vi "Get Positions.vi"(8 "error in":errorcluster, 11 "Stage VISA in":refnum<visa-resource-name>) -> (0 "error out":errorcluster, 2 "Stage current position":dbl[](array[numeric]), 3 "Stage VISA out":refnum<visa-resource-name>)   [LabVIEW 2017]
panel:
  # "X"
  # "Y"
  # "Z"
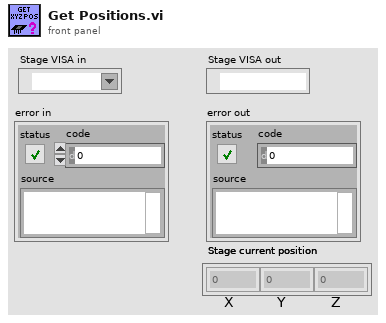
[diagram p1: front panel]
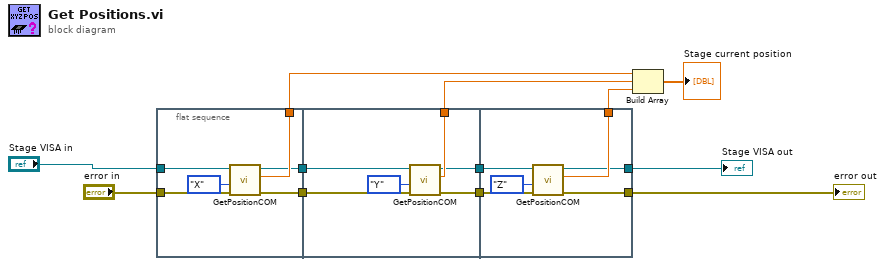
[diagram p0: block diagram]
diagram:
  n1 = flat-sequence {
    tunnel: "error in" -> [w17]
    tunnel: [w18] -> w10
    tunnel: [w16] -> w7
    tunnel: [w15] -> w3
    tunnel: "Stage VISA in" -> [w14]
    tunnel: [w22] -> w6
    tunnel: [w24] -> w9
    tunnel: w10 -> [w23]
    tunnel: [w21] -> w4
    tunnel: w3 -> [w20]
    tunnel: [w29] -> w11
    tunnel: w9 -> [w30]
    tunnel: [w28] -> w5
    tunnel: [w27] -> w1
    tunnel: w4 -> [w26]
    frame #0 {
      n2 = call "GetPositionCOM.vi"("error in"=w17, "Axis"=enum16{"X", "Y", "Z"}."X", "VISA resource name"=w14) -> ("error out"=w18:errorcluster, "Position (mm)"=w16:dbl, "VISA resource name out"=w15:refnum<visa-resource-name>)  [unwired: 6 in]
    }
    frame #1 {
      n3 = call "GetPositionCOM.vi"("error in"=w23, "Axis"=enum16{"X", "Y", "Z"}."Y", "VISA resource name"=w20) -> ("error out"=w24:errorcluster, "Position (mm)"=w22:dbl, "VISA resource name out"=w21:refnum<visa-resource-name>)  [unwired: 6 in]
    }
    frame #2 {
      n4 = call "GetPositionCOM.vi"("error in"=w30, "Axis"=enum16{"X", "Y", "Z"}."Z", "VISA resource name"=w26) -> ("error out"=w29:errorcluster, "Position (mm)"=w28:dbl, "VISA resource name out"=w27:refnum<visa-resource-name>)  [unwired: 6 in]
    }
  }
  n5 = Build Array(w7, w6, w5) -> (→"Stage current position":dbl[])
  "error out" <- w11
  "Stage VISA out" <- w1
